vi "Manage UI and GFG states during settings file edit.vi"(7 "Commands":T2, 8 "Error In":errorcluster, 9 "Command String IN":string, 10 "UI control refnums":T1) -> (0 "Error Out":errorcluster)   [LabVIEW 2012]
doc: "SciScan 1.2 160622"
uses:
  Update Scan Settings_Commands.ctl
  Custom Controls and Typedefs/Macro_MD_UI Control Refnums.ctl
  Custom Controls and Typedefs/Delete Button.ctl
  Custom Controls and Typedefs/Edit Button.ctl
  Custom Controls and Typedefs/Timing Estimate Cluster.ctl
  CommonResource VIs/Timing/Timing Indicator.ctl
  Custom Controls and Typedefs/Load from PSM Button.ctl
  CommonResource VIs/UI Control and Indicator properties_Commands.ctl
  GFG/GFGfpRefGet.vi
  GFG/GFG library.lvlib
panel:
  # "(hh:mm:ss)"
  # "(hh:mm:ss)"
  # "(hh:mm:ss)"
  # "(hh:mm:ss)"
  # "(hh:mm:ss)"
  # "(hh:mm:ss)"
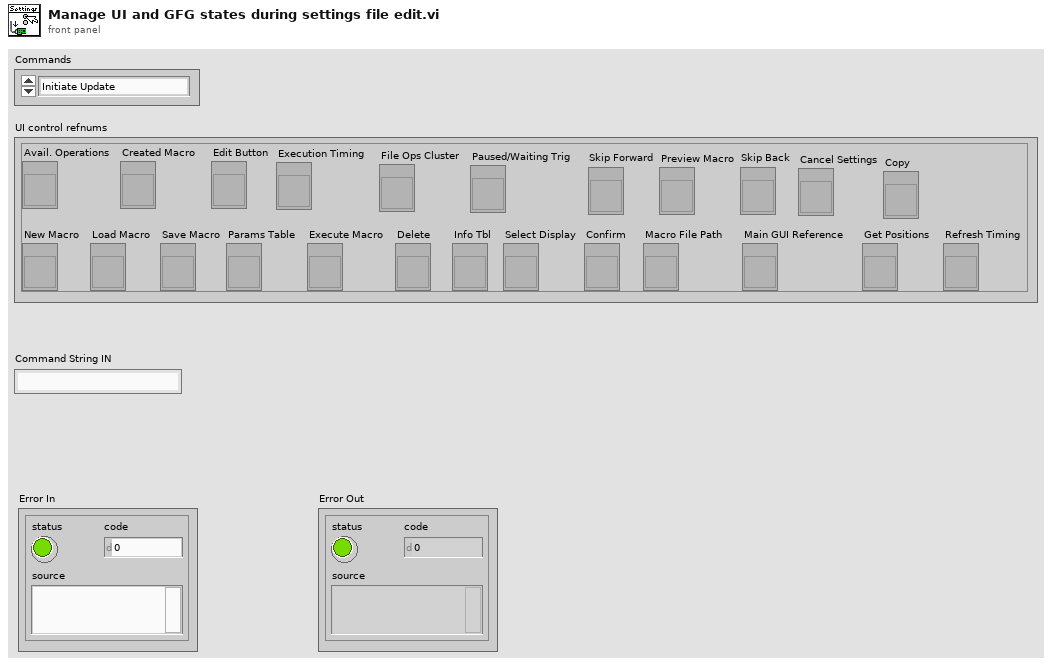
[diagram p1: front panel]
types:
  T1 = typedef "Macro_MD_UI Control Refnums.ctl" = cluster{"Avail. Operations":refnum<vi>, "Created Macro":refnum<vi>, "Load Macro":refnum<vi>, "Save Macro":refnum<vi>, "Params Table":refnum<vi>, "Delete":refnum<vi>, "Edit Button":refnum<vi>, "Execute Macro":refnum<vi>, "Info Tbl":refnum<vi>, "Execution Timing":refnum<vi>, "Select Display":refnum<vi>, "File Ops Cluster":refnum<vi>, "Paused/Waiting Trig":refnum<vi>, "Confirm":refnum<vi>, "New Macro":refnum<vi>, "Preview Macro":refnum<vi>, "Skip Forward":refnum<vi>, "Skip Back":refnum<vi>, "Macro File Path":refnum<vi>, "Main GUI Reference":refnum<vi>, "Cancel Settings":refnum<vi>, "Get Positions":refnum<vi>, "Copy":refnum<vi>, "Refresh Timing":refnum<vi>}
  T2 = typedef "Update Scan Settings_Commands.ctl" = enum16{"Initiate Update", "Finalise Update"}
  T3 = enum32{"Invalid", "Default", "Floating", "Floating/Auto-Hide", "Modal"}
  T4 = typedef "UI Control and Indicator properties_Commands.ctl" = enum16{"Enable", "Disable", "Disable and Grey", "Make Visible", "Make Invisible"}
  T5 = enum8{"Enabled", "Disabled", "Disabled and Grayed Out"}
  T6 = cluster{"WaveformChartRef":refnum<vi>, "DigitalRef":refnum<vi>, "ArrayRef":refnum<vi>, "TabControlRef":refnum<vi>, "EnumRef":refnum<vi>, "RingRef":refnum<vi>, "BooleanRef":refnum<vi>, "KnobRef":refnum<vi>, "SlideRef":refnum<vi>, "PathRef":refnum<vi>, "StringRef":refnum<vi>, "ComboBox":refnum<vi>, "WaveformGraphRef":refnum<vi>}
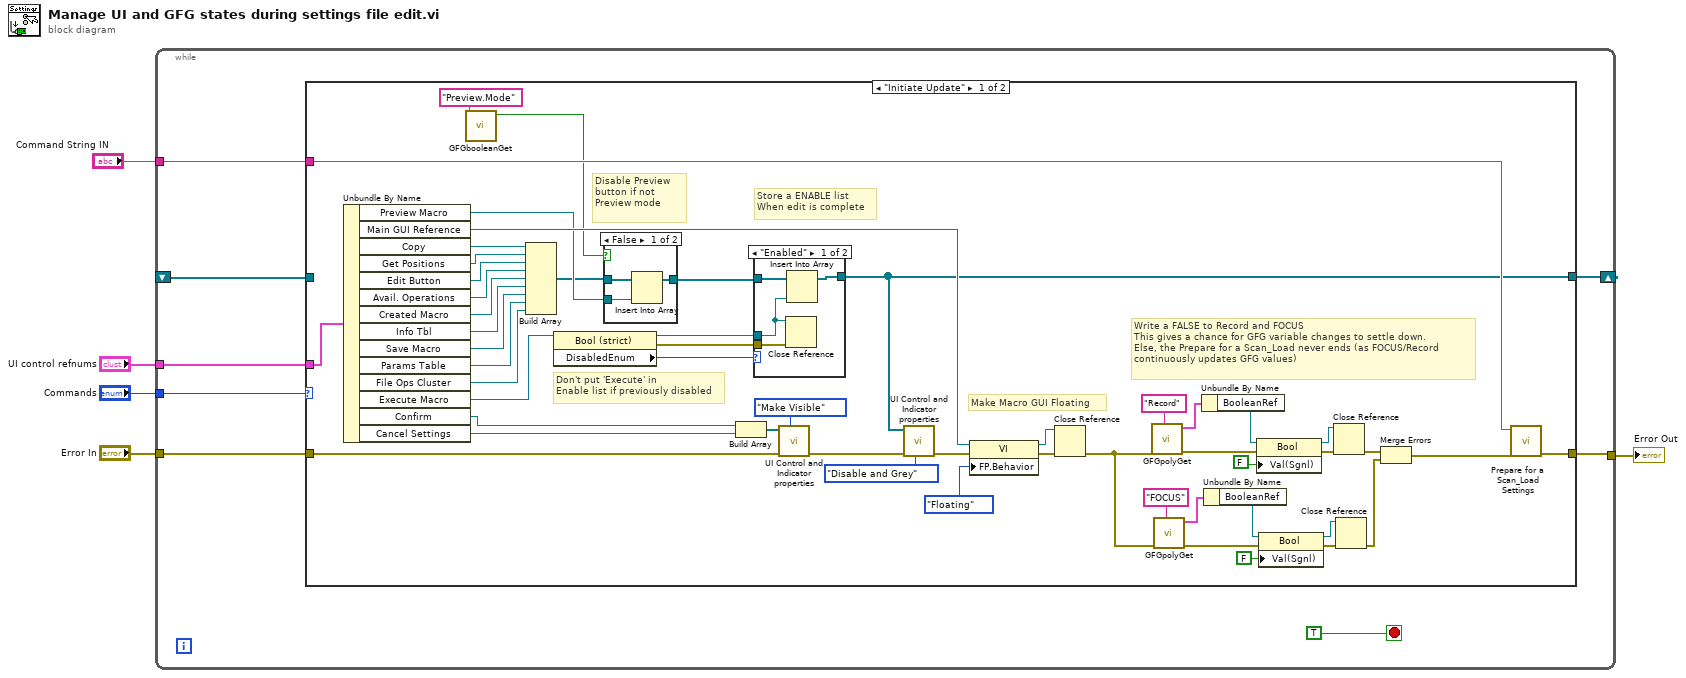
[diagram p0: block diagram]
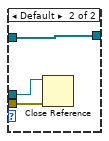
[diagram p3: hidden frame]
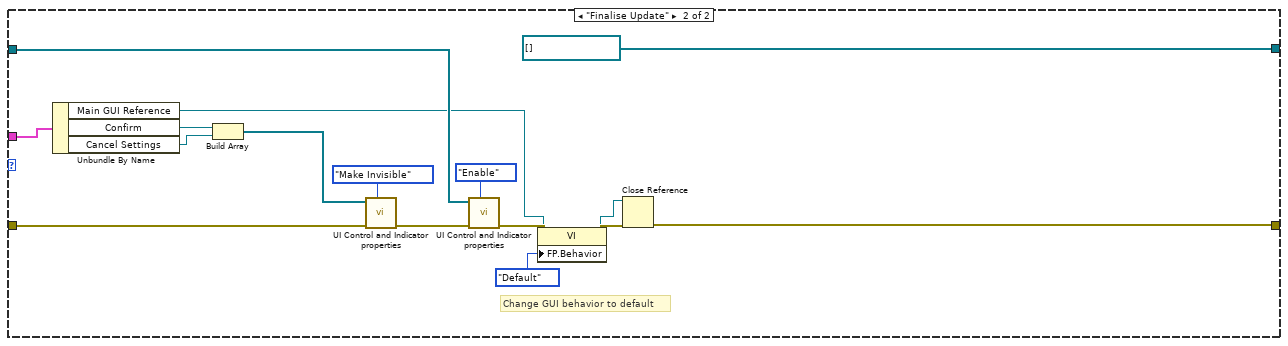
[diagram p4: hidden frame]
diagram:
  n1 = while {
    tunnel: "Commands" -> [w12]
    tunnel: "Error In" -> [w11]
    tunnel: "UI control refnums" -> [w10]
    tunnel: [w9] -> w2
    shift-right: [w8] -> _
    shift-left: _ -> [w7]
    tunnel: "Command String IN" -> [w6]
    stop <- TRUE stop-if-true
    n2 = case shown="\"Initiate Update\"" w12 {
      tunnel: w11 -> [w44 w77]
      tunnel: w10 -> [w65 w92]
      tunnel: [w41 w79] -> w9
      tunnel: [w14 refnum<vi>[] []] -> w8
      tunnel: w7 -> [_ w86]
      tunnel: w6 -> [w25 _]
      frame "Initiate Update" {
        # "Don't put 'Execute' in\nEnable list if previously disabled"
        # "Store a ENABLE list\nWhen edit is complete"
        # "Disable Preview button if not Preview mode"
        # "Write a FALSE to Record and FOCUS\nThis gives a chance for GFG variable changes to settle down.\nElse, the Prepare for a Scan_Load never ends (as FOCUS/Record continuously updates GFG values)"
        # "Make Macro GUI Floating"
        n3 = Unbundle By Name(w65) -> ("Preview Macro"=w17:refnum<vi>, "Main GUI Reference"=w49:refnum<vi>, "Copy"=w20:refnum<vi>, "Get Positions"=w21:refnum<vi>, "Edit Button"=w42:refnum<vi>, "Avail. Operations"=w50:refnum<vi>, "Created Macro"=w51:refnum<vi>, "Info Tbl"=w59:refnum<vi>, "Save Macro"=w58:refnum<vi>, "Params Table"=w57:refnum<vi>, "File Ops Cluster"=w56:refnum<vi>, "Execute Macro"=w55:refnum<vi>, "Confirm"=w64:refnum<vi>, "Cancel Settings"=w43:refnum<vi>)
        n4 = call "GFGbooleanGet.vi"("Variable Name in"="Preview.Mode") -> ("Boolean Value OUT"=w18:bool)  [unwired: 9 in, 1 out]
        n5 = Build Array(w20, w21, w42, w50, w51, w59, w58, w57, w56) -> (w16:refnum<vi>[])
        n6 = property class="Bool (strict)"(reference=w55) -> (reference out=w53:refnum<vi>, error out=w52:errorcluster, "DisabledEnum"=w54:T5)  [unwired: 1 in]
        n7 = case shown="False" w18 {
          tunnel: w17 -> [w66 _]
          tunnel: w16 -> [w68 w69]
          tunnel: [w67 w69] -> w15
          frame False {
            n8 = Insert Into Array(array=w68, new element=w66) -> (w67:refnum<vi>[])  [unwired: 1 in]
          }
          frame True {
          }
        }
        n9 = Build Array(w64, w43) -> (w62:refnum<vi>[])
        n10 = case shown="\"Enabled\"" w54 {
          tunnel: w15 -> [w73 w76]
          tunnel: w53 -> [w71 w74]
          tunnel: [w72 w76] -> w14
          tunnel: w52 -> [w70 w75]
          frame "Enabled" {
            n11 = Close Reference(reference=w71, error in (no error)=w70) -> ()  [unwired: 1 out]
            n12 = Insert Into Array(array=w73, new element=w71) -> (w72:refnum<vi>[])  [unwired: 1 in]
          }
          frame Default {
            n13 = Close Reference(reference=w74, error in (no error)=w75) -> ()  [unwired: 1 out]
          }
        }
        n14 = call "UI Control and Indicator properties.vi"("Enable Command"=UI_Control_and_Indicator_properties_Commands."Make Visible", "Error In"=w44, "Control Refnums"=w62) -> ("Error Out"=w60:errorcluster)  [unwired: 8 in]
        n15 = call "UI Control and Indicator properties.vi"("Enable Command"=UI_Control_and_Indicator_properties_Commands."Disable and Grey", "Error In"=w60, "Control Refnums"=w14) -> ("Error Out"=w48:errorcluster)  [unwired: 8 in]
        n16 = property class="VI"(reference=w49, error in=w48, "FP.Behavior"=T3."Floating" ("Front Panel Window:Behavior")) -> (reference out=w45:refnum<vi>, error out=w46:errorcluster)
        n17 = Close Reference(reference=w45, error in (no error)=w46) -> (error out=w26:errorcluster)
        n18 = call-poly "GFGpolyGet.vi"("error in (no error)"=w26, "Variable Name in"="Record") -> ("error out"=w35:errorcluster, "output cluster"=w36:T6)  [unwired: 8 in]
        n19 = call-poly "GFGpolyGet.vi"("error in (no error)"=w26, "Variable Name in"="FOCUS") -> ("error out"=w32:errorcluster, "output cluster"=w31:T6)  [unwired: 8 in]
        n20 = Unbundle By Name(w36) -> ("BooleanRef"=w40:refnum<vi>)
        n21 = Unbundle By Name(w31) -> ("BooleanRef"=w27:refnum<vi>)
        n22 = property class="Bool"(reference=w40, error in=w35, "Val(Sgnl)"=FALSE) -> (reference out=w37:refnum<vi>, error out=w38:errorcluster)
        n23 = property class="Bool"(reference=w27, error in=w32, "Val(Sgnl)"=FALSE) -> (reference out=w30:refnum<vi>, error out=w29:errorcluster)
        n24 = Close Reference(reference=w37, error in (no error)=w38) -> (error out=w24:errorcluster)
        n25 = Close Reference(reference=w30, error in (no error)=w29) -> (error out=w23:errorcluster)
        n26 = Merge Errors(w24, w23) -> (w22:errorcluster)
        n27 = call "Prepare for a Scan_Load Settings.vi"("error in (no error)"=w22, "Command IN"=w25) -> ("error out"=w41:errorcluster)  [unwired: 9 in]
      }
      frame "Finalise Update" {
        # "Change GUI behavior to default"
        n28 = Unbundle By Name(w92) -> ("Main GUI Reference"=w80:refnum<vi>, "Confirm"=w91:refnum<vi>, "Cancel Settings"=w78:refnum<vi>)
        n29 = Build Array(w91, w78) -> (w89:refnum<vi>[])
        n30 = call "UI Control and Indicator properties.vi"("Enable Command"=UI_Control_and_Indicator_properties_Commands."Make Invisible", "Error In"=w77, "Control Refnums"=w89) -> ("Error Out"=w87:errorcluster)  [unwired: 8 in]
        n31 = call "UI Control and Indicator properties.vi"("Enable Command"=UI_Control_and_Indicator_properties_Commands."Enable", "Error In"=w87, "Control Refnums"=w86) -> ("Error Out"=w81:errorcluster)  [unwired: 8 in]
        n32 = property class="VI"(reference=w80, error in=w81, "FP.Behavior"=T3."Default" ("Front Panel Window:Behavior")) -> (reference out=w83:refnum<vi>, error out=w84:errorcluster)
        n33 = Close Reference(reference=w83, error in (no error)=w84) -> (error out=w79:errorcluster)
      }
    }
  }
  "Error Out" <- w2
